vi "ArduinoFinal.vi"(8 "Error In":errorcluster, 10 "Knob":u8(knob)=4 scale=4.0..10.0, 11 "Serial Port":refnum<visa-resource-name>="COM4") -> (0 "Error Out":errorcluster, 2 "Response":u8[](array[numeric]))   [LabVIEW 2015]
uses:
  <vilib>/MakerHub/LINX/Public/Utilities/Open Serial.vi
  <vilib>/MakerHub/LINX/LMH-LINX.lvlib
panel:
  in  "Degrees Per Step":u8=30
  in  "Start Button":bool
  in  "?":bool
  out "Input Array":u8[](array[numeric])
  out "Delay (Hz)":u32
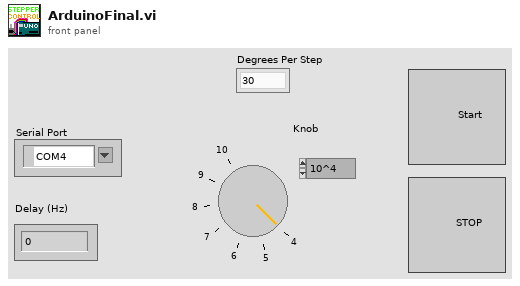
[diagram p1: front panel]
types:
  T1 = typedef "LMH-LINX.lvlib/LINX Ref.ctl" = cluster{"IO":T2, "Interface":T3, "LINX Device Config":T4}
  T2 = typedef "LMH-LINX.lvlib/Platform.ctl" = enum16{"Remote", "Local"}
  T3 = typedef "LMH-LINX.lvlib/Interface.ctl" = enum16{"Serial", "TCP"}
  T4 = typedef "LMH-LINX.lvlib/Device.lvlib/LINX Device Config.ctl" = cluster{"Interface":T3, "COM Port":refnum<visa-resource-name>, "TCP Configuration":T5, "Device Family":u8, "Device ID":u8, "Device Name":string, "TCP Ref":refnum<k5>, "Channels":T6}
  T5 = typedef "LMH-LINX.lvlib/Device.lvlib/TCP Config.ctl" = cluster{"IP Address":string, "Port":u16}
  T6 = typedef "LMH-LINX.lvlib/Channels.ctl" = cluster{"DI":u8[], "DO":u8[], "AI":u8[], "AO":u8[], "PWM":u8[], "QE":u8[], "UART":u8[], "I2C 2":u8[], "SPI":u8[], "CAN":u8[], "Servo":u8[], "AI Ref (V)":dbl, "AI Resolution (Bits)":u8, "AO Ref (V)":dbl, "AO Resolution (Bits)":u8}
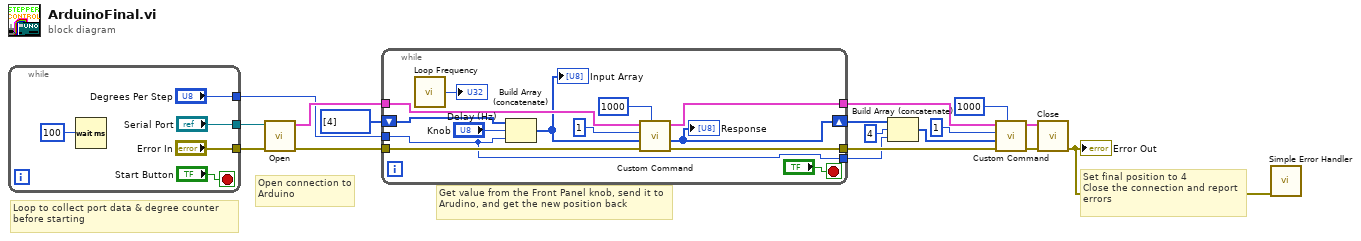
[diagram p0: block diagram]
diagram:
  # "Loop to collect port data & degree counter before starting"
  # "Set final position to 4\nClose the connection and report errors"
  # "Get value from the Front Panel knob, send it to Arudino, and get the new position back"
  # "Open connection to Arduino"
  n1 = while {
    tunnel: ["Serial Port"] -> w17
    tunnel: ["Error In"] -> w14
    tunnel: ["Degrees Per Step"] -> w2
    stop <- "Start Button" stop-if-true
    n2 = Wait (ms)(milliseconds to wait=u32 100) -> ()  [unwired: 1 out]
  }
  n3 = call-poly <vilib>:"Open.vi"("Error In"=w14, "Serial Port"=w17) -> ("Error Out"=w15:errorcluster, "LINX Resource"=w16:T1)  [unwired: 7 in, 1 out]
  n4 = while {
    tunnel: w16 -> [w32]
    tunnel: [w35] -> w12
    tunnel: [w33] -> w11
    tunnel: w15 -> [w34]
    shift-right: [w31] -> w4
    shift-left: u8[] [4] ("Response") -> [w30]
    tunnel: w2 -> [w23]
    tunnel: [w23] -> w1
    stop <- "?" stop-if-true
    n5 = call <vilib>:"Loop Frequency.vi"() -> ("Loop Rate (Hz)"=→"Delay (Hz)":u32)
    n6 = Build Array (concatenate)(w30, "Knob", w23) -> (w27:u8[])
    "Input Array" <- w27
    n7 = call <vilib>:"Custom Command.vi"("Timeout (100 ms)"=1000, "Error In"=w34, "Data"=w27, "Custom Command Number"=u16 1, "LINX Resource"=w32) -> ("Error Out"=w33:errorcluster, "Response"=w31:u8[], "LINX Resource"=w35:T1)  [unwired: 3 in, 1 out]
    "Response" <- w31
  }
  n8 = Build Array (concatenate)(w4, u8 4, w1) -> (w7:u8[])
  n9 = call <vilib>:"Custom Command.vi"("Timeout (100 ms)"=1000, "Error In"=w11, "Data"=w7, "Custom Command Number"=u16 1, "LINX Resource"=w12) -> ("Error Out"=w10:errorcluster, "LINX Resource"=w9:T1)  [unwired: 3 in, 2 out]
  n10 = call <vilib>:"Close.vi"("Error In"=w10, "LINX Resource"=w9) -> ("Error Out"=w13:errorcluster)  [unwired: 9 in]
  "Error Out" <- w13
  n11 = call <vilib>:"Simple Error Handler.vi"("error in (no error)"=w13) -> ()  [unwired: 4 in, 5 out]
